vi "FPGA Direct IO Template.vi"() -> ()   [LabVIEW 2017, in "NI_Robotics_Starter Kit Direct IO_FPGA.lvlib"]
uses:
  <vilib>/robotics/Starter Kit/FPGA Direct IO/NI_Robotics_Starter Kit Direct IO_FPGA.lvlib
panel:
  in  "FPGA LED":bool
  in  "DCmotor_1_direct":bool
  in  "DCmotor_0_direct":bool
  in  "servo_0_direct":bool
  in  "ModB/AO0":fxp<+/-,20,5> format="%.17g"
  in  "ModB/AO1":fxp<+/-,20,5> format="%.17g"
  in  "ModB/AO2":fxp<+/-,20,5> format="%.17g"
  in  "ModB/AO3":fxp<+/-,20,5> format="%.17g"
  out "ModA/AI0":fxp<+/-,26,5> format="%.23g"
  out "ModA/AI1":fxp<+/-,26,5> format="%.23g"
  out "ModA/AI2":fxp<+/-,26,5> format="%.23g"
  out "ModA/AI3":fxp<+/-,26,5> format="%.23g"
  out "ModA/AI7":fxp<+/-,26,5> format="%.23g"
  out "ModA/AI6":fxp<+/-,26,5> format="%.23g"
  out "ModA/AI5":fxp<+/-,26,5> format="%.23g"
  out "ModA/AI4":fxp<+/-,26,5> format="%.23g"
  out "ModA/AI9":fxp<+/-,26,5> format="%.23g"
  out "ModA/AI8":fxp<+/-,26,5> format="%.23g"
  in  "DCmotor_1_PWM":T1={"period (us)"=20000, "pulse width (us)"=1500}
  in  "DCmotor_0_PWM":T1={"period (us)"=20000, "pulse width (us)"=1500}
  in  "servo_0_PWM":T1={"period (us)"=20000, "pulse width (us)"=1500}
  in  "Port7/DIO0_PWM":T1={"period (us)"=20000, "pulse width (us)"=1500}
  in  "Port7/DIO1_PWM":T1={"period (us)"=20000, "pulse width (us)"=1500}
  in  "Port7/DIO2_PWM":T1={"period (us)"=20000, "pulse width (us)"=1500}
  in  "Port7/DIO3_PWM":T1={"period (us)"=20000, "pulse width (us)"=1500}
  in  "Port3/DIO0":bool
  in  "Port3/DIO0_write":bool
  in  "Port3/DIO1":bool
  in  "Port3/DIO1_write":bool
  in  "Port3/DIO2":bool
  in  "Port3/DIO2_write":bool
  in  "Port3/DIO3":bool
  in  "Port3/DIO3_write":bool
  in  "Port3/DIO4":bool
  in  "Port3/DIO4_write":bool
  in  "Port3/DIO5":bool
  in  "Port3/DIO5_write":bool
  in  "Port3/DIO6":bool
  in  "Port3/DIO6_write":bool
  in  "Port3/DIO7":bool
  in  "Port3/DIO7_write":bool
  in  "Port3/DIO8":bool
  in  "Port3/DIO8_write":bool
  in  "Port3/DIO9":bool
  in  "Port3/DIO9_write":bool
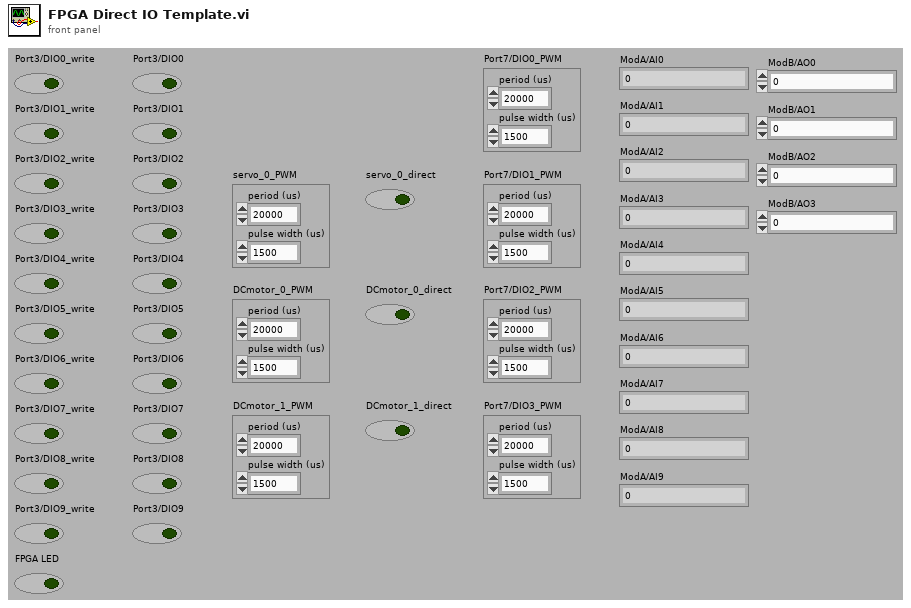
[diagram p1: front panel]
types:
  T1 = cluster{"period (us)":u32, "pulse width (us)":u32}
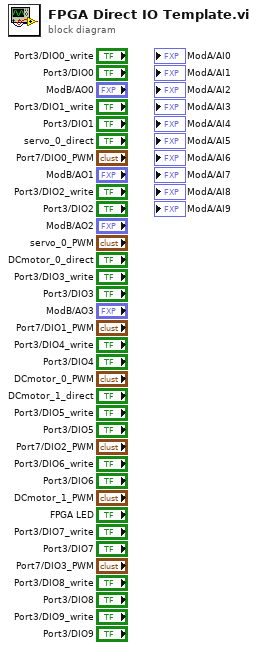
[diagram p0: block diagram]
diagram:
